vi "get_ave_value.vi"(9 "number_of_values":u16, 11 "value_in (convert to sgl)":sgl) -> (3 "ave_value":sgl)   [LabVIEW 2020]
panel:
  out "sum":sgl
  out "count":u16
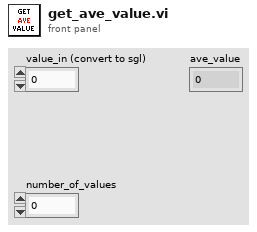
[diagram p1: front panel]
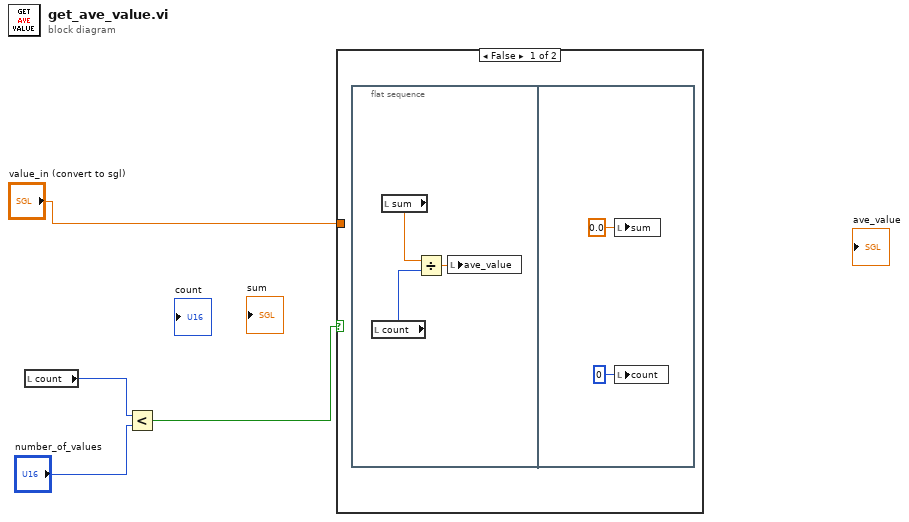
[diagram p0: block diagram]
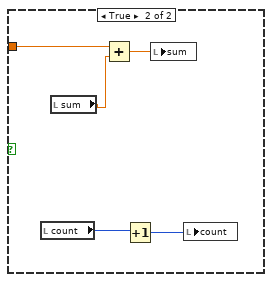
[diagram p2: hidden frame]
diagram:
  n1 = local read "count"() -> (w3:u16)
  n2 = Less?(x=w3, y="number_of_values") -> (x < y?=w1:bool)
  n3 = case shown="False" w1 {
    tunnel: "value_in (convert to sgl)" -> [_ w10]
    frame False {
      n4 = flat-sequence {
        frame #0 {
          n5 = local read "count"() -> (w5:u16)
          n6 = local read "sum"() -> (w6:sgl)
          n7 = Divide(x=w6, y=w5) -> (x/y=w7:sgl)
          n8 = local write "ave_value"(w7) -> ()
        }
        frame #1 {
          n9 = local write "sum"(sgl 0.0 ("sum")) -> ()
          n10 = local write "count"(u16 0 ("count")) -> ()
        }
      }
    }
    frame True {
      n11 = local read "count"() -> (w12:u16)
      n12 = local read "sum"() -> (w13:sgl)
      n13 = Add(x=w10, y=w13) -> (x+y=w14:sgl)
      n14 = Increment(x=w12) -> (x+1=w11:u16)
      n15 = local write "sum"(w14) -> ()
      n16 = local write "count"(w11) -> ()
    }
  }
